vi "Run Test.vi"(0 "TestProcessor in":refnum<class "TestProcessor.lvclass">, 5 "Command Directors":refnum<class "CommandDirector.lvclass">[](array[class]), 7 "Wait Time":u32 caption="ms" step=1, 9 "Results Notifier":refnum<notifier>, 11 "error in (no error)":errorcluster, 12 "Handle Injections":bool) -> (4 "TestProcessor out":refnum<class "TestProcessor.lvclass">, 15 "error out":errorcluster)   [LabVIEW 2023, in "HAF.lvlib" / "TestProcessor.lvclass"]
doc: "Processes all the passed Command Directors until they complete. This member will respond to events to Pause, Resume and Stop. Results will be notified on the Notification Queue.\n\nIf the array of Command Directors is empty, it will use the existing Command Directors, assuming that they have been added individually. Obviously, if there are no Command Directors the test finishes immediately."
uses:
  TestProcessor.lvclass
  ReadCommand/ReadCommand.lvclass
  CommandDirector/CommandDirector.lvclass
  TestProcessor.lvclass/TestProcessor.ctl
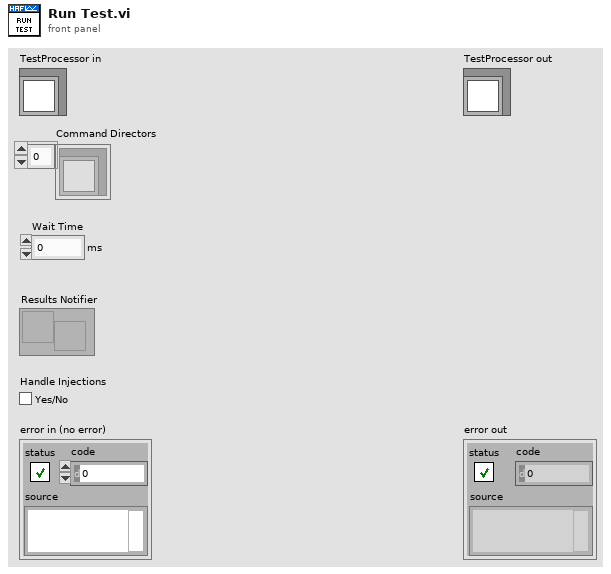
[diagram p1: front panel]
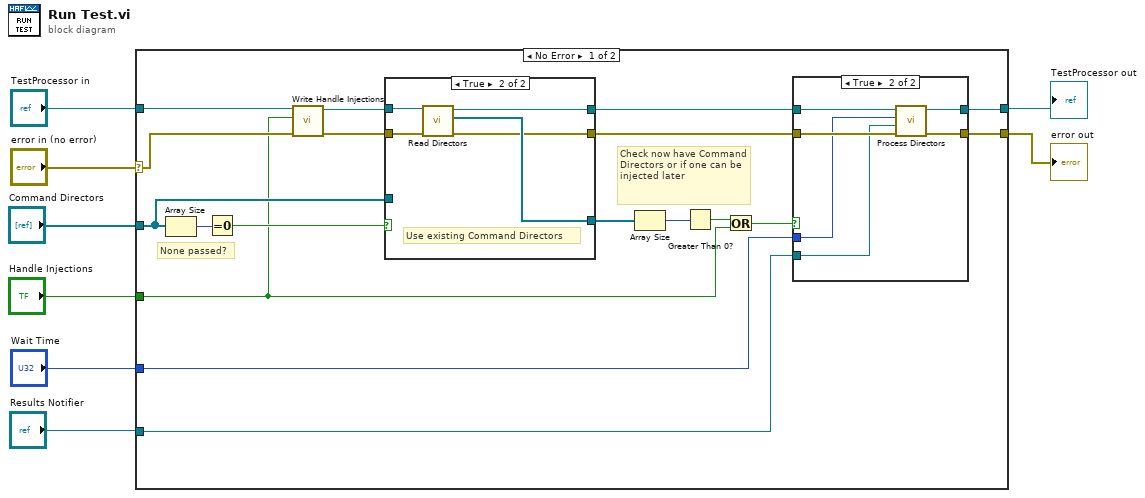
[diagram p0: block diagram]
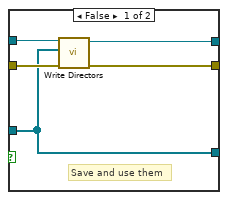
[diagram p3: hidden frame]
diagram:
  n1 = case shown="No Error" "error in (no error)" {
    selector: "error in (no error)" -> [w11 w46]
    tunnel: [w18 w46] -> w2
    tunnel: [w19 w45] -> w3
    tunnel: "TestProcessor in" -> [w13 w45]
    tunnel: "Command Directors" -> [w24 _]
    tunnel: "Wait Time" -> [w21 _]
    tunnel: "Results Notifier" -> [w20 _]
    tunnel: "Handle Injections" -> [w9 _]
    frame No Error {
      # "Check now have Command Directors or if one can be injected later"
      # "None passed?"
      n2 = Array Size(array=w24) -> (size(s)=w26:i32)
      n3 = Equal To 0?(x=w26) -> (x = 0?=w25:bool)
      n4 = call-dynamic "Write Handle Injections.vi"("error in (no error)"=w11, "Handle Injections"=w9, "TestProcessor in"=w13) -> ("error out"=w10:errorcluster, "TestProcessor out"=w12:refnum<class "TestProcessor.lvclass">)  [unwired: 7 in]
      n5 = case shown="True" w25 {
        tunnel: w10 -> [w38 w44]
        tunnel: w12 -> [w39 w43]
        tunnel: w24 -> [w36 _]
        tunnel: [w36 w42] -> w17
        tunnel: [w37 w41] -> w22
        tunnel: [w35 w40] -> w23
        frame False {
          # "Save and use them"
          n6 = call-dynamic "Write Directors.vi"("error in (no error)"=w38, "Directors"=w36, "TestProcessor in"=w39) -> ("error out"=w37:errorcluster, "TestProcessor out"=w35:refnum<class "TestProcessor.lvclass">)  [unwired: 7 in]
        }
        frame True {
          # "Use existing Command Directors"
          n7 = call-dynamic "Read Directors.vi"("error in (no error)"=w44, "TestProcessor in"=w43) -> ("error out"=w41:errorcluster, "Directors"=w42:refnum<class "CommandDirector.lvclass">[], "TestProcessor out"=w40:refnum<class "TestProcessor.lvclass">)  [unwired: 7 in]
        }
      }
      n8 = Array Size(array=w17) -> (size(s)=w16:i32)
      n9 = Greater Than 0?(x=w16) -> (x > 0?=w15:bool)
      n10 = Or(x=w15, y=w9) -> (x .or. y?=w14:bool)
      n11 = case shown="True" w14 {
        tunnel: w23 -> [w28 w34]
        tunnel: w22 -> [w27 w33]
        tunnel: w21 -> [_ w32]
        tunnel: w20 -> [_ w31]
        tunnel: [w28 w30] -> w19
        tunnel: [w27 w29] -> w18
        frame False {
          # "Do nothing, there are no Command Directors"
        }
        frame True {
          n12 = call-dynamic "Process Directors.vi"("error in (no error)"=w33, "Results Notifier"=w31, "Wait Time"=w32, "TestProcessor in"=w34) -> ("error out"=w29:errorcluster, "TestProcessor out"=w30:refnum<class "TestProcessor.lvclass">)  [unwired: 6 in]
        }
      }
    }
    frame Error {
    }
  }
  "error out" <- w2
  "TestProcessor out" <- w3
